vi "Handle Response.vi"(6 "Last Toggle-Bit":bool, 7 "ICommunicate":refnum<class "ICommunicate.lvclass">, 8 "Error In":errorcluster, 9 "Response":refnum<class "CANopen Response Message.lvclass">, 10 "Service Data Object":refnum<class "Service Data Object.lvclass">, 11 "reference in":refnum<class "SDO Manager.lvclass">) -> (0 "Error Out":errorcluster, 1 "Value":u8[](array[numeric]), 2 "Success?":bool, 3 "reference out":refnum<class "SDO Manager.lvclass">)   [LabVIEW 2024]
uses:
  SDO Manager.lvclass/SDO Manager.ctl
  CANopen Response/CANopen Response Message.lvclass
  CANopen Message/CANopen Message.lvclass
  2f0e94ff-a21a-4829-93b9-c94b55c38f4a.vi
  213bcf54-0e5d-4ef6-a5ce-d33c9996973b.vi
  SDO Manager.lvclass
  9a973c79-e5b2-48d0-8cef-0ce60df170f2.vi
  Service Data Object/Service Data Object.lvclass
  95763af5-508b-45a0-9dd1-44b0f543477d.vi
  HAL/Source/Interfaces/ICommunicate/ICommunicate.lvclass
panel:
  out "size":u32
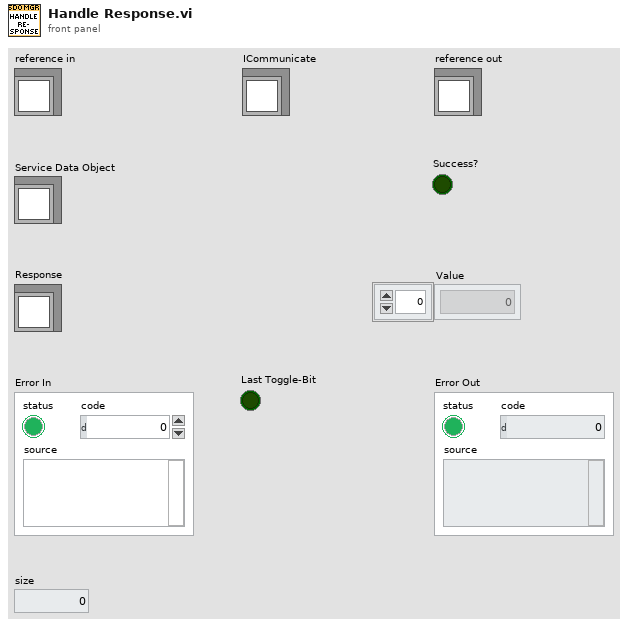
[diagram p1: front panel]
types:
  T1 = typedef "CANopen Response Message.lvclass/Server Command Specifier.ctl" = enum8{"Upload Segment Response", "Download Segment Response", "Initiate Upload Response", "Initiate Download Response", "Heartbeat", "Block Download"}
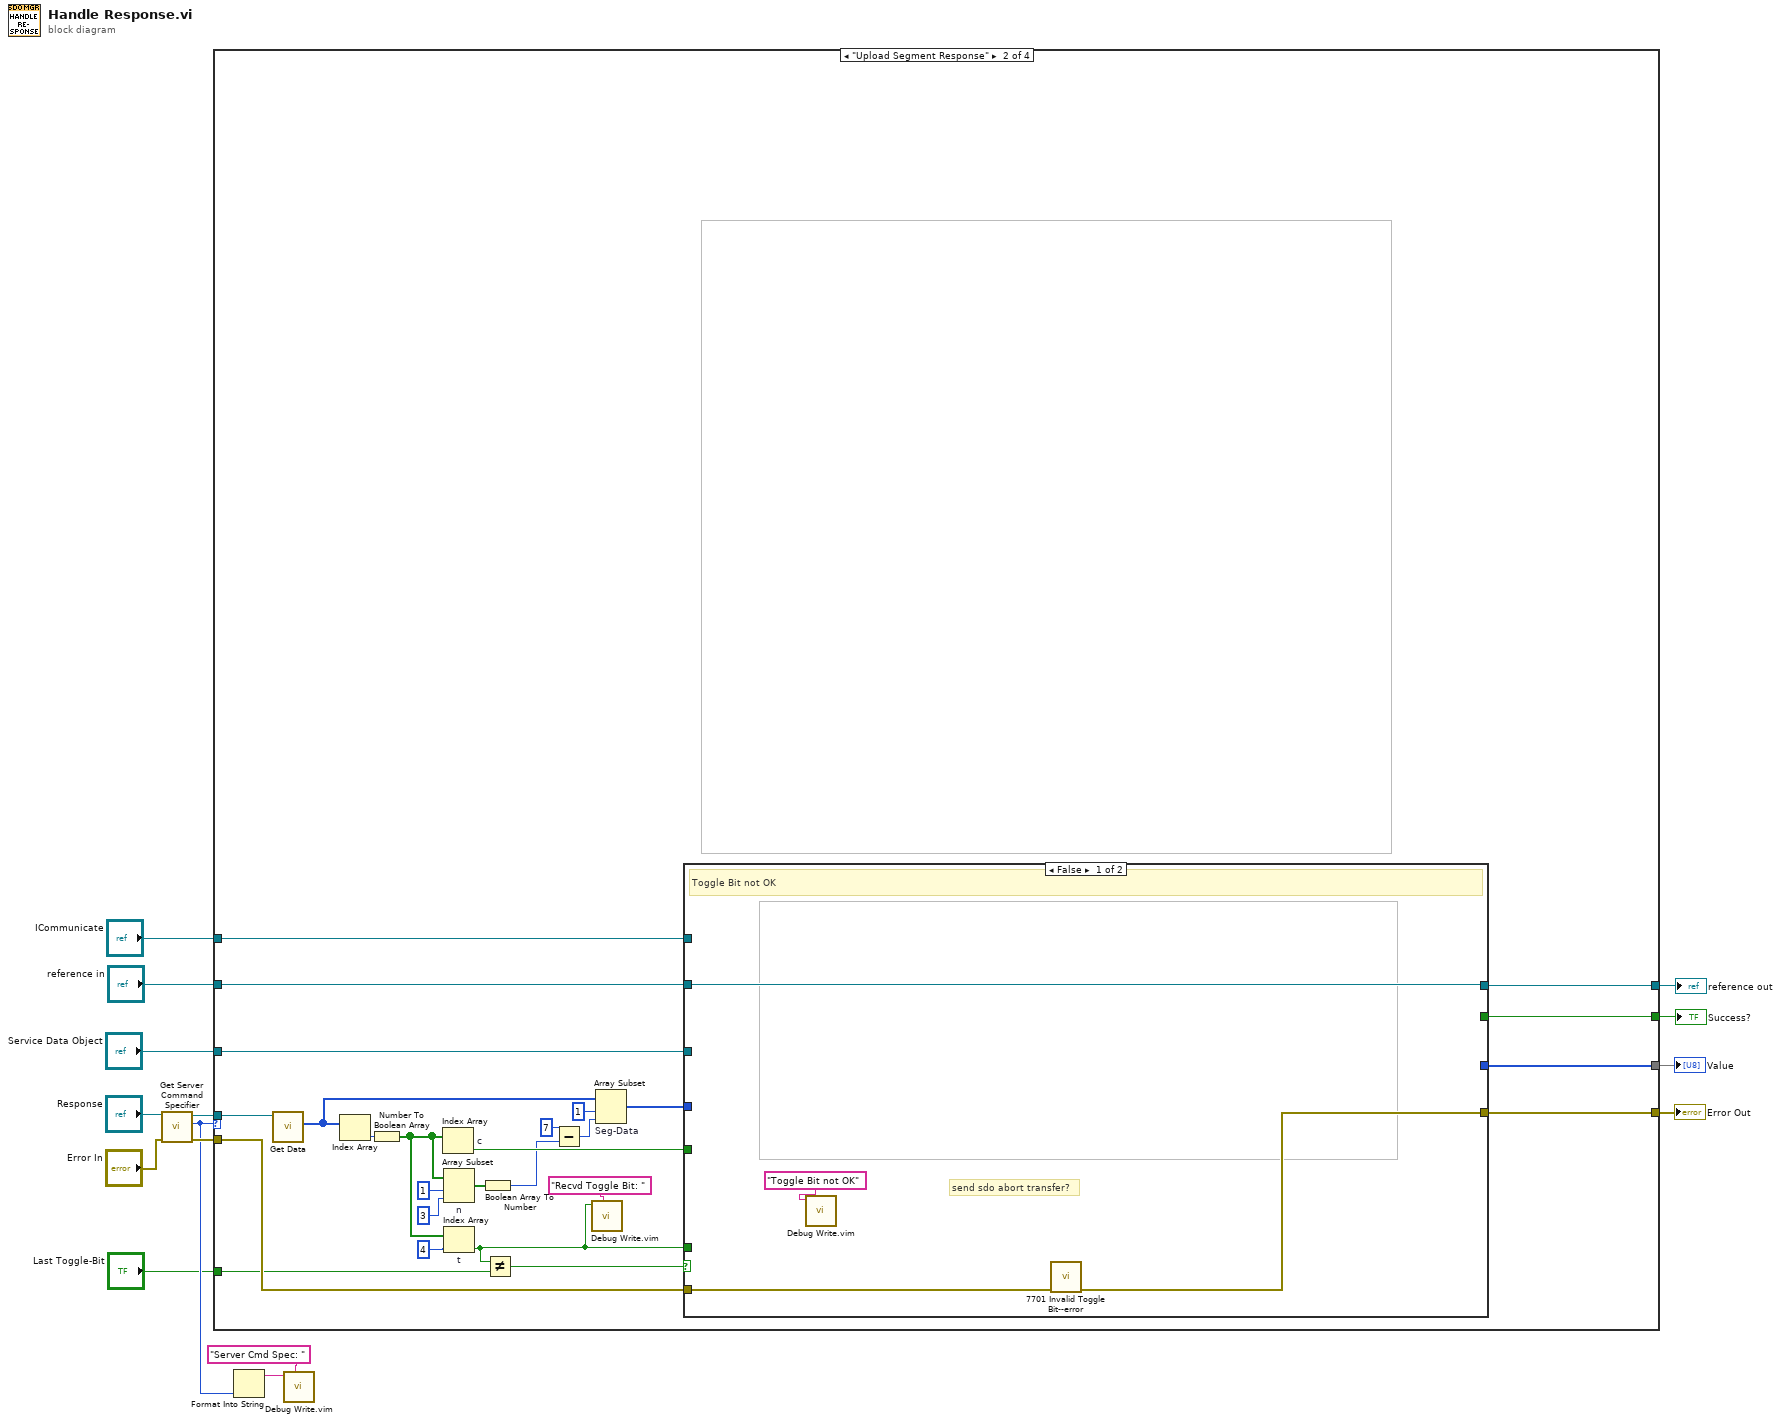
[diagram p0: block diagram]
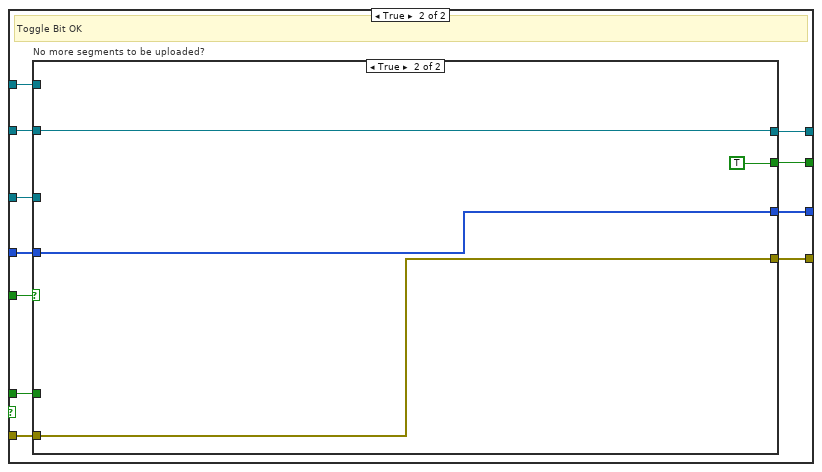
[diagram p3: hidden frame]
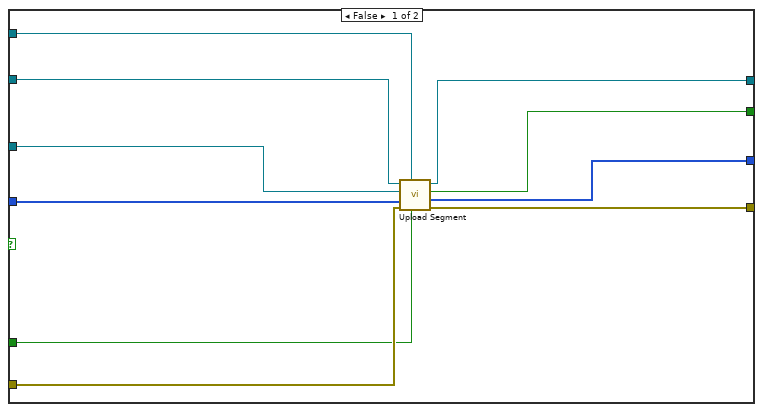
[diagram p4: hidden frame]
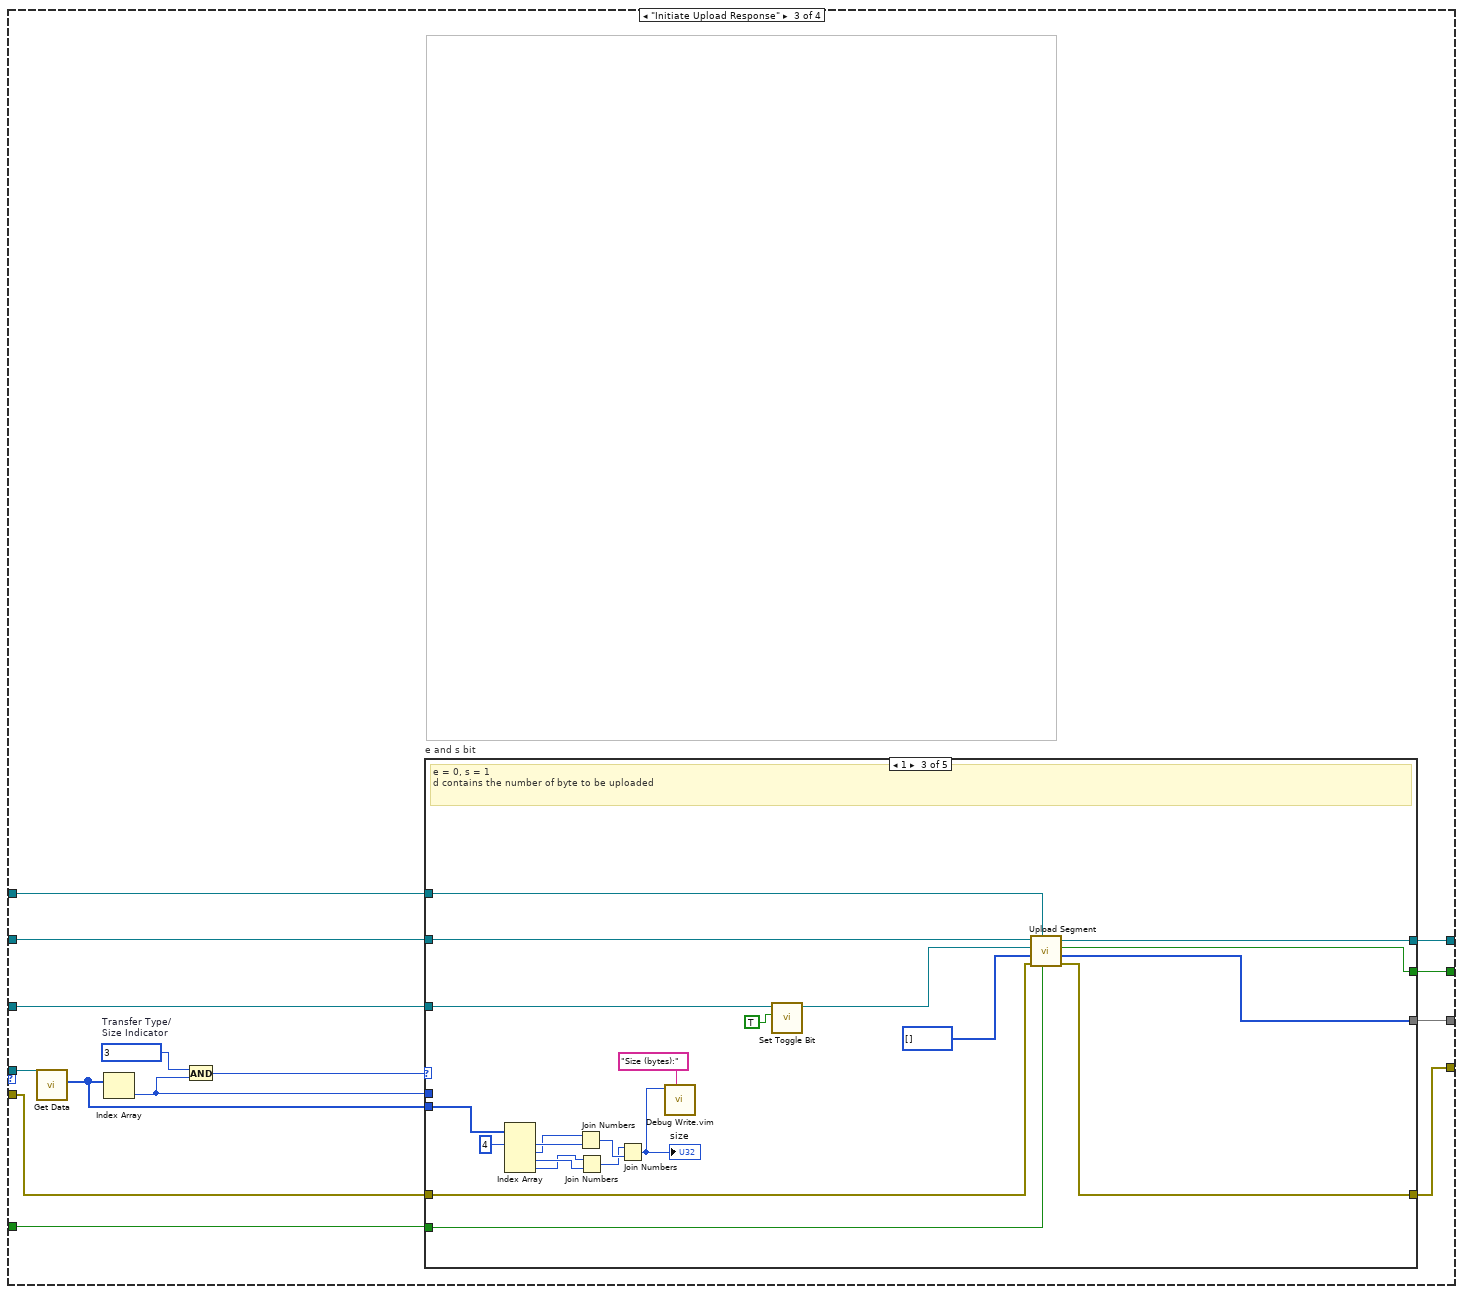
[diagram p5: hidden frame]
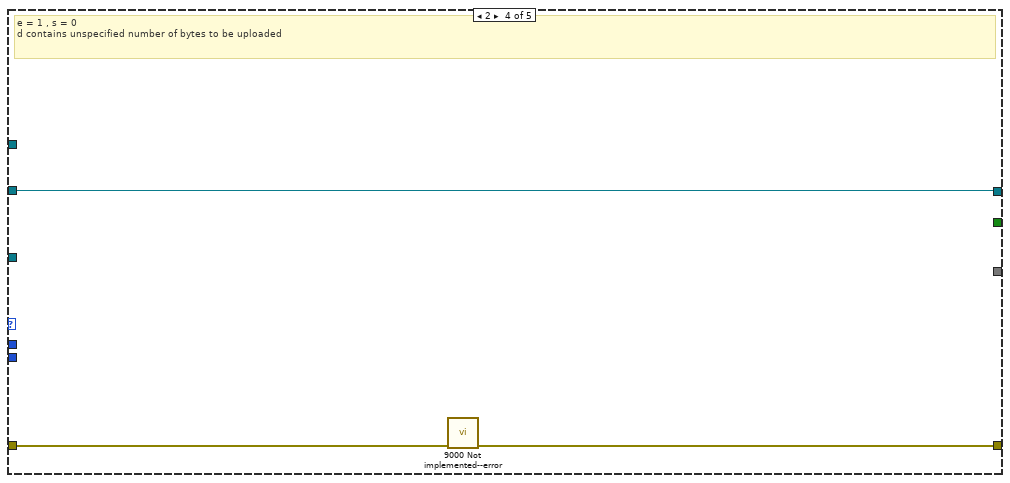
[diagram p8: hidden frame]
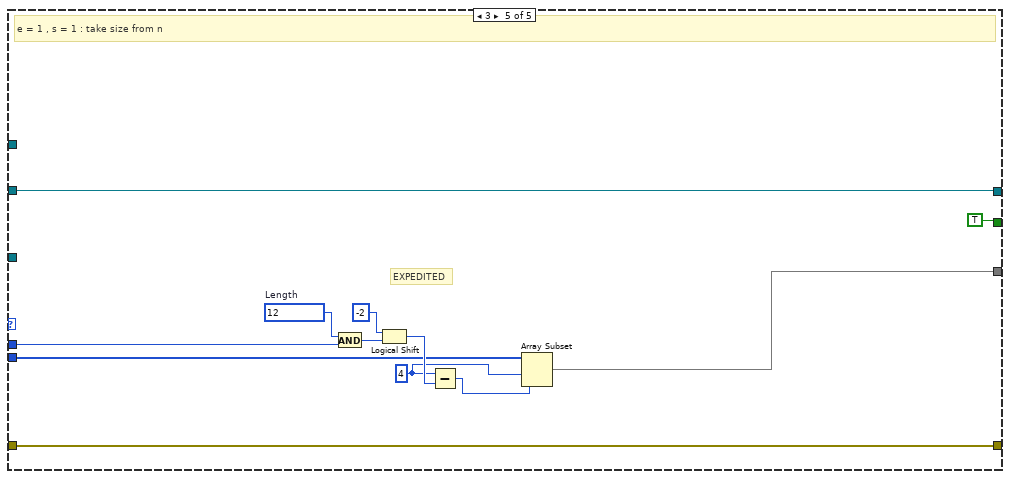
[diagram p9: hidden frame]
diagram:
  n1 = call-dynamic "Get Server Command Specifier.vi"("error in"="Error In", "CANopen Response in"="Response") -> ("error out"=w7:errorcluster, "Server Command Specifier"=w3:T1, "CANopen Response out"=w9:refnum<class "CANopen Response Message.lvclass">)  [unwired: 7 in]
  n2 = case shown="\"Upload Segment Response\"" w3 {
    tunnel: [w17 w32 w76 w128] -> w15
    tunnel: "reference in" -> [w16 w35 w79 w129]
    tunnel: [w16 w31 w78 w129] -> w13
    tunnel: "ICommunicate" -> [_ w36 w80 _]
    tunnel: w9 -> [_ w43 w82 _]
    tunnel: [_ w37 w81 _] -> w8
    tunnel: w7 -> [w17 w33 w77 w128]
    tunnel: "Service Data Object" -> [_ w34 w75 _]
    tunnel: [_ w30 w74 _] -> w5
    tunnel: "Last Toggle-Bit" -> [_ w27 w73 _]
    frame Default {
    }
    frame "Upload Segment Response" {
      n3 = call "Get Data.vi"("CANopen Message in"=w43) -> ("Data"=w22:u8[])  [unwired: 8 in, 2 out]
      n4 = Index Array(array=w22) -> (element=w42:u8)  [unwired: 1 in]
      n5 = Number To Boolean Array(number=w42) -> (Boolean array=w29:bool[])
      n6 = Index Array "c"(array=w29) -> (element=w38:bool)  [unwired: 1 in]
      n7 = Array Subset "n"(array=w29, index=1, length=3) -> (w39:bool[])
      n8 = Index Array "t"(array=w29, index=4) -> (element=w18:bool)
      n9 = Boolean Array To Number(Boolean array=w39) -> (number=w21:u32)
      n10 = Not Equal?(x=w18, y=w27) -> (x != y?=w26:bool)
      n11 = Subtract(x=7 ("index"), y=w21) -> (x-y=w23:u32)
      n12 = call "Debug Write.vim"("prefix (\"\")"="Recvd Toggle Bit: " ("prefix (\"\")"), "value"=w18) -> ()  [unwired: 9 in, 1 out]
      n13 = Array Subset "Seg-Data"(array=w22, index=1, length=w23) -> (w20:u8[])
      n14 = case "Toggle Bit Check" shown="False" w26 {
        tunnel: w38 -> [_ w58]
        tunnel: [_ w57] -> w37
        tunnel: w36 -> [_ w56]
        tunnel: w35 -> [w47 w55]
        tunnel: w34 -> [_ w54]
        tunnel: w33 -> [w46 w53]
        tunnel: [w45 w52] -> w32
        tunnel: [w47 w51] -> w31
        tunnel: [_ w50] -> w30
        tunnel: w18 -> [_ w49]
        tunnel: w20 -> [_ w48]
        frame False {
          # "send sdo abort transfer?"
          # "Toggle Bit not OK"
          n15 = call "Debug Write.vim"("value"="Toggle Bit not OK" ("prefix (\"\")")) -> ()  [unwired: 10 in, 1 out]
          n16 = call "7701 Invalid Toggle Bit--error.vi"("error in"=w46) -> ("error out"=w45:errorcluster)  [unwired: 10 in]
        }
        frame True {
          # "Toggle Bit OK"
          n17 = case "No more segments to be uploaded?" shown="True" w58 {
            tunnel: w48 -> [w60 w72]
            tunnel: [w61 w72] -> w57
            tunnel: w56 -> [w67 _]
            tunnel: w55 -> [w68 w71]
            tunnel: w54 -> [w66 _]
            tunnel: w53 -> [w65 w70]
            tunnel: [w64 w70] -> w52
            tunnel: [w63 w71] -> w51
            tunnel: [w62 TRUE ("Success?")] -> w50
            tunnel: w49 -> [w59 _]
            frame False {
              n18 = call "Upload Segment.vi"("Last Toggle Bit"=w59, "ICommunicate"=w67, "error in"=w65, "Concetenated Value"=w60, "Service Data Object"=w66, "SDO Manager in"=w68) -> ("error out"=w64:errorcluster, "Concetenated Value out"=w61:u8[], "Success?"=w62:bool, "SDO Manager out"=w63:refnum<class "SDO Manager.lvclass">)  [unwired: 2 in]
            }
            frame True {
            }
          }
        }
      }
    }
    frame "Initiate Upload Response" {
      w86 = u8 3  # Transfer Type/ Size Indicator
      n19 = call "Get Data.vi"("CANopen Message in"=w82) -> ("Data"=w83:u8[])  [unwired: 8 in, 2 out]
      n20 = Index Array(array=w83) -> (element=w84:u8)  [unwired: 1 in]
      n21 = And(x=w86, y=w84) -> (x .and. y?=w85:u8)
      n22 = case "e and s bit" shown="1" w85 {
        tunnel: w84 -> [_ _ _ _ w127]
        tunnel: w83 -> [_ _ w112 _ w122]
        tunnel: [_ _ w99 _ w119] -> w81
        tunnel: w80 -> [_ _ w98 _ _]
        tunnel: w79 -> [w88 w89 w103 w115 w118]
        tunnel: [w88 w89 w102 w115 w118] -> w78
        tunnel: w77 -> [w87 w90 w104 w114 w117]
        tunnel: [w87 w90 w101 w113 w117] -> w76
        tunnel: w75 -> [_ _ w93 _ _]
        tunnel: [_ _ w100 _ TRUE ("Success?")] -> w74
        tunnel: w73 -> [_ _ w94 _ _]
        frame Default {
          # "INVALID - CAN'T BE REACHED"
        }
        frame 0 {
          # "e = 0, s = 0 d is reserved for further use"
        }
        frame 1 {
          # "e = 0, s = 1\nd contains the number of byte to be uploaded"
          n23 = Index Array(array=w112, index #1=4 ("index")) -> (element #1=w110:u8, element #2=w109:u8, element #3=w108:u8, element #4=w107:u8)  [unwired: 3 in]
          n24 = Join Numbers(hi=w109, lo=w110) -> ((hi.lo)=w106:u16)
          n25 = Join Numbers(hi=w107, lo=w108) -> ((hi.lo)=w105:u16)
          n26 = Join Numbers(hi=w105, lo=w106) -> ((hi.lo)=w97:u32)
          "size" <- w97
          n27 = call "Debug Write.vim"("prefix (\"\")"="Size (bytes):" ("prefix (\"\")"), "value"=w97) -> ()  [unwired: 9 in, 1 out]
          n28 = call "Set Toggle Bit.vi"("Toggle Bit"=TRUE, "Service Data Object in"=w93) -> ("Service Data Object out"=w92:refnum<class "Service Data Object.lvclass">)  [unwired: 9 in]
          n29 = call "Upload Segment.vi"("Last Toggle Bit"=w94, "ICommunicate"=w98, "error in"=w104, "Concetenated Value"=u8[] [] ("Accumulated Value"), "Service Data Object"=w92, "SDO Manager in"=w103) -> ("error out"=w101:errorcluster, "Concetenated Value out"=w99:u8[], "Success?"=w100:bool, "SDO Manager out"=w102:refnum<class "SDO Manager.lvclass">)  [unwired: 2 in]
        }
        frame 2 {
          # "e = 1 , s = 0 \nd contains unspecified number of bytes to be uploaded"
          n30 = call "9000 Not implemented--error.vi"("error in"=w114) -> ("error out"=w113:errorcluster)  [unwired: 10 in]
        }
        frame 3 {
          w120 = 4 ("index")
          w126 = u8 12  # Length
          # "EXPEDITED"
          # "e = 1 , s = 1 : take size from n"
          n31 = And(x=w126, y=w127) -> (x .and. y?=w125:u8)
          n32 = Logical Shift(y=i16 -2, x=w125) -> (x << y=w123:u8)
          n33 = Subtract(x=w120, y=w123) -> (x-y=w121:i32)
          n34 = Array Subset(array=w122, index=w120, length=w121) -> (w119:u8[])
        }
      }
    }
    frame "Download Segment Response" {
    }
  }
  "Error Out" <- w15
  "reference out" <- w13
  "Value" <- w8
  "Success?" <- w5
  n35 = Format Into String(w3) -> (resulting string=w2:string)  [unwired: 3 in, 1 out]
  n36 = call "Debug Write.vim"("prefix (\"\")"="Server Cmd Spec: " ("prefix (\"\")"), "value"=w2) -> ()  [unwired: 9 in, 1 out]
